vi "Gyro Init.vi"(8 "error in (no error)":errorcluster, 11 "I2C Information Out":T1) -> (0 "error out":errorcluster, 3 "FPGA Information Out":T1)   [LabVIEW 2012]
uses:
  <vilib>/IEDriver/SPIandI2C/Host/I2C/I2C Host.lvlib
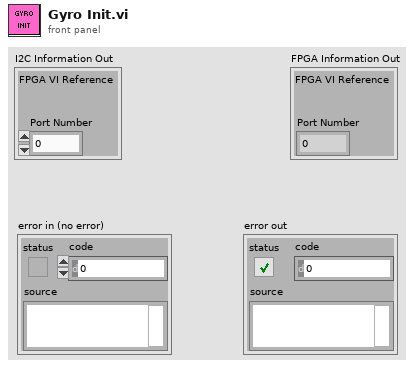
[diagram p1: front panel]
types:
  T1 = cluster{"FPGA VI Reference":refnum<k20>, "Port Number":u8}
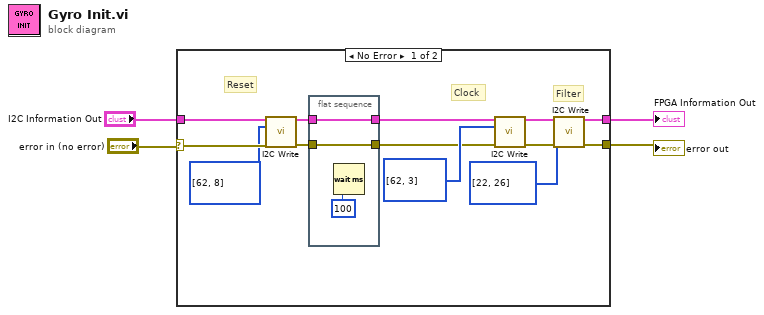
[diagram p0: block diagram]
diagram:
  n1 = case shown="No Error" "error in (no error)" {
    selector: "error in (no error)" -> [w10 w21]
    tunnel: "I2C Information Out" -> [w11 w22]
    tunnel: [w13 w22] -> w3
    tunnel: [w12 w21] -> w1
    frame No Error {
      # "Filter"
      # "Clock"
      # "Reset"
      n2 = call <vilib>:"I2C Write.vi"("FPGA Information In"=w11, "Data"=u8[] [62, 8], "error in (no error)"=w10) -> ("FPGA Information Out"=w8:T1, "error out"=w7:errorcluster)  [unwired: 11 in]
      n3 = flat-sequence {
        tunnel: w8 -> [w20]
        tunnel: w7 -> [w19]
        tunnel: [w20] -> w6
        tunnel: [w19] -> w5
        frame #0 {
          n4 = Wait (ms)(milliseconds to wait=u32 100) -> ()  [unwired: 1 out]
        }
      }
      n5 = call <vilib>:"I2C Write.vi"("FPGA Information In"=w6, "Data"=u8[] [62, 3], "error in (no error)"=w5) -> ("FPGA Information Out"=w15:T1, "error out"=w16:errorcluster)  [unwired: 11 in]
      n6 = call <vilib>:"I2C Write.vi"("FPGA Information In"=w15, "Data"=u8[] [22, 26], "error in (no error)"=w16) -> ("FPGA Information Out"=w13:T1, "error out"=w12:errorcluster)  [unwired: 11 in]
    }
    frame Error {
    }
  }
  "FPGA Information Out" <- w3
  "error out" <- w1
